vi "FR GUI Connections.vi"() -> ()   [LabVIEW 2020]
panel:
  out "actual connection":picture
  in  "hide":bool
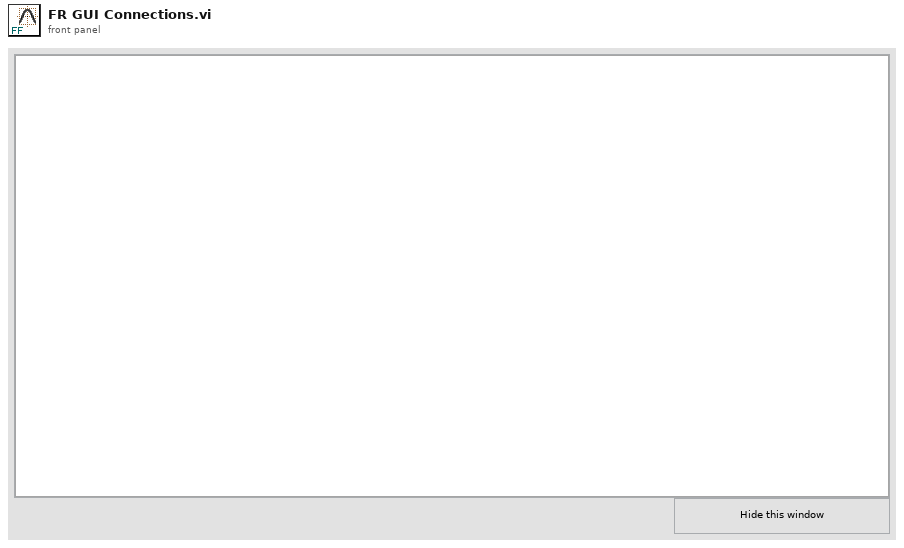
[diagram p1: front panel]
types:
  T1 = typedef "imagedata.ctl" = cluster{"image type":i32, "image depth":i32, "image":u8[], "mask":u8[], "colors":u32[], "Rectangle":cluster{"left":i16, "top":i16, "right":i16, "bottom":i16}}
  T2 = enum32{"Invalid", "Standard", "Closed", "Hidden", "Minimized", "Maximized"}
  T3 = typedef "LVRectTypeDef.ctl" = cluster{"Left":i16, "Top":i16, "Right":i16, "Bottom":i16}
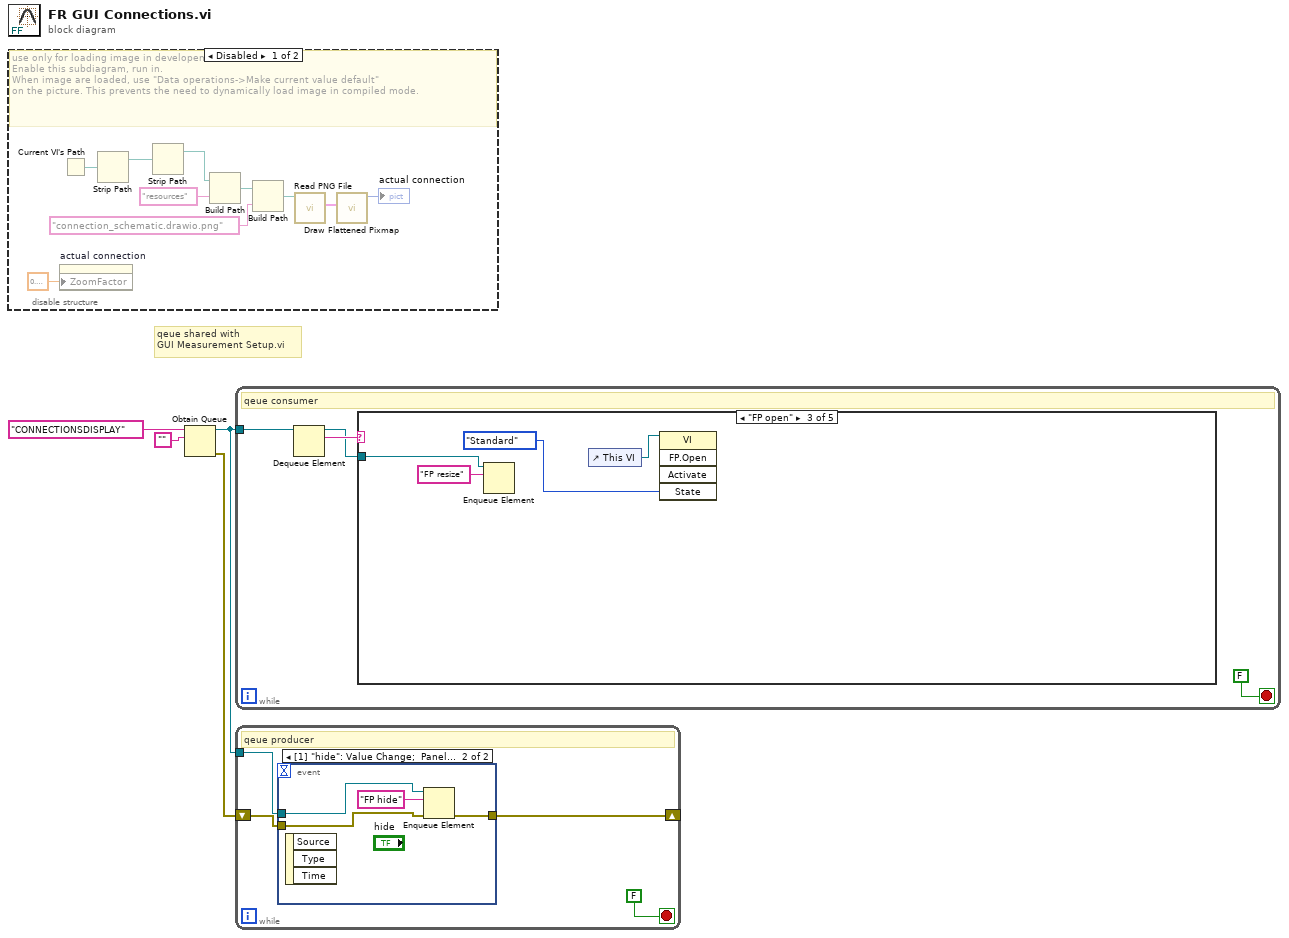
[diagram p0: block diagram]
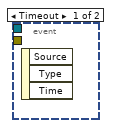
[diagram p2: hidden frame]
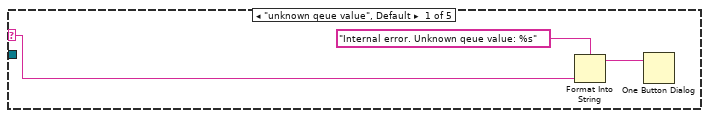
[diagram p3: hidden frame]
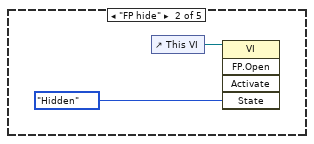
[diagram p4: hidden frame]
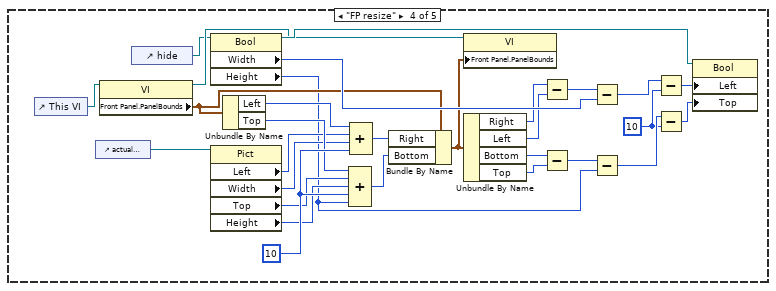
[diagram p5: hidden frame]
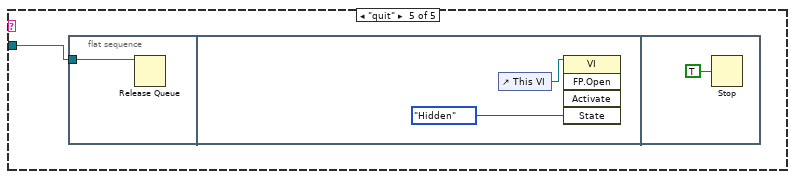
[diagram p6: hidden frame]
diagram:
  # "qeue shared with\nGUI Measurement Setup.vi"
  n1 = disable-structure shown="Disabled" {
    frame Disabled {
      # "use only for loading image in developement mode.\nEnable this subdiagram, run in.\nWhen image are loaded, use \"Data operations->Make current value default\" \non the picture. This prevents the need to dynamically load image in compiled mode."
      n2 = property on="actual connection" class="Pict"("ZoomFactor"=sgl 0.4 ("Zoom Factor")) -> ()  [unwired: 2 in, 2 out]
      n3 = Current VI's Path() -> (path=w14:path)
      n4 = Strip Path(path=w14) -> (stripped path=w13:path)  [unwired: 1 out]
      n5 = Strip Path(path=w13) -> (stripped path=w12:path)  [unwired: 1 out]
      n6 = Build Path(base path=w12, name or relative path="resources") -> (appended path=w10:path)
      n7 = Build Path(base path=w10, name or relative path="connection_schematic.drawio.png") -> (appended path=w7:path)
      n8 = call <vilib>:"Read PNG File.vi"("path to PNG file"=w7) -> ("image data"=w8:T1)  [unwired: 8 in, 2 out]
      n9 = call <vilib>:"Draw Flattened Pixmap.vi"("image data"=w8) -> ("new picture"=→"actual connection":picture)  [unwired: 8 in]
    }
    frame Enabled {
    }
  }
  n10 = Obtain Queue(name (unnamed)="CONNECTIONSDISPLAY", element data type="" ("data (can be any type)")) -> (queue out=w1:refnum<queue>, error out=w2:errorcluster)  [unwired: 3 in, 1 out]
  n11 = while {
    tunnel: w1 -> [w17]
    stop <- FALSE stop-if-true
    # "qeue consumer"
    n12 = Dequeue Element(queue=w17) -> (queue out=w15:refnum<queue>, element=w16:string)  [unwired: 2 in, 2 out]
    n13 = case shown="\"FP open\"" w16 {
      selector: w16 -> [w19 _ _ _ _]
      tunnel: w15 -> [_ _ w24 _ w57]
      frame "unknown qeue value", Default {
        n14 = Format Into String(format string="Internal error. Unknown qeue value: %s", w19) -> (resulting string=w21:string)  [unwired: 2 in, 1 out]
        n15 = One Button Dialog(message=w21) -> ()  [unwired: 1 in, 1 out]
      }
      frame "FP hide" {
        n16 = control-ref of="This VI"() -> (w22:refnum<vi>)
        n17 = invoke class="VI" method="FP.Open"(reference=w22, "State"=T2."Hidden") -> ()  [unwired: 3 in, 5 out]
      }
      frame "FP open" {
        n18 = Enqueue Element(queue=w24, element="FP resize") -> ()  [unwired: 2 in, 3 out]
        n19 = control-ref of="This VI"() -> (w26:refnum<vi>)
        n20 = invoke class="VI" method="FP.Open"(reference=w26, "State"=T2."Standard") -> ()  [unwired: 3 in, 5 out]
      }
      frame "FP resize" {
        w37 = u32 10 ("value")
        w42 = u32 10 ("y")
        n21 = control-ref of="This VI"() -> (w44:refnum<vi>)
        n22 = control-ref of="actual connection"() -> (w28:refnum<vi>)
        n23 = property class="VI"(reference=w44) -> (reference out=w43:refnum<vi>, "Front Panel.PanelBounds"=w40:T3)  [unwired: 1 in, 1 out]
        n24 = control-ref of="hide"() -> (w29:refnum<vi>)
        n25 = property class="Bool"(reference=w29) -> (reference out=w56:refnum<vi>, "Width"=w55:u32, "Height"=w31:u32)  [unwired: 1 in, 1 out]
        n26 = property class="Pict"(reference=w28) -> ("Left"=w33:i32, "Width"=w34:u32, "Top"=w32:i32, "Height"=w36:u32)  [unwired: 1 in, 2 out]
        n27 = Unbundle By Name(w40) -> ("Left"=w41:i16, "Top"=w35:i16)
        n28 = Compound Arithmetic op=ADD(w35, w32, w36, w37, w31) -> (w38:u32)
        n29 = Compound Arithmetic op=ADD(w41, w33, w34, w37) -> (w39:u32)
        n30 = Bundle By Name(cluster=w40, "Right"=w39, "Bottom"=w38) -> (w30:T3)
        n31 = property class="VI"(reference=w43, "Front Panel.PanelBounds"=w30) -> ()  [unwired: 1 in, 2 out]
        n32 = Unbundle By Name(w30) -> ("Right"=w50:i16, "Left"=w49:i16, "Bottom"=w53:i16, "Top"=w51:i16)
        n33 = Subtract(x=w50, y=w49) -> (x-y=w54:i16)
        n34 = Subtract(x=w53, y=w51) -> (x-y=w52:i16)
        n35 = Subtract(x=w54, y=w55) -> (x-y=w48:u32)
        n36 = Subtract(x=w52, y=w31) -> (x-y=w47:u32)
        n37 = Subtract(x=w48, y=w42) -> (x-y=w46:u32)
        n38 = Subtract(x=w47, y=w42) -> (x-y=w45:u32)
        n39 = property class="Bool"(reference=w56, "Left"=w46, "Top"=w45) -> ()  [unwired: 1 in, 2 out]
      }
      frame "quit" {
        n40 = flat-sequence {
          tunnel: w57 -> [w58]
          frame #0 {
            n41 = Release Queue(queue=w58) -> ()  [unwired: 2 in, 3 out]
          }
          frame #1 {
            n42 = control-ref of="This VI"() -> (w59:refnum<vi>)
            n43 = invoke class="VI" method="FP.Open"(reference=w59, "State"=T2."Hidden") -> ()  [unwired: 3 in, 5 out]
          }
          frame #2 {
            n44 = Stop(stop? (T)=TRUE) -> ()
          }
        }
      }
    }
  }
  n45 = while {
    shift-right: [w64] -> _
    shift-left: w2 -> [w65]
    tunnel: w1 -> [w63]
    stop <- FALSE stop-if-true
    # "qeue producer"
    n46 = event shown="[1] \"hide\": Value Change;  Panel Close" {
      selector: _ -> [_ _]
      dyn-events: _ -> [_ _]
      timeout: _ -> [_ _]
      tunnel: w65 -> [_ w68]
      tunnel: [_ w67] -> w64
      tunnel: w63 -> [_ w66]
      event Timeout {
        n47 = event-data() -> ()  [unwired: 1 in, 3 out]
      }
      event "hide": Value Change; Panel Close {
        n48 = event-data() -> ()  [unwired: 1 in, 3 out]
        n49 = Enqueue Element(queue=w66, element="FP hide", error in (no error)=w68) -> (error out=w67:errorcluster)  [unwired: 1 in, 2 out]
      }
    }
  }
